vi "example.vi"() -> ()   [LabVIEW 2021]
uses:
  QR Code Reader.lvclass
  C:/Users/HEP/Documents/GitHub/Gantry/UCSB-Gantry-HEP-main/Classes/Controller/Camera/Camera.lvclass
  <vilib>/vision/Image Controls.llb/IMAQ Image.ctl
  <vilib>/vision/Instrument.llb/Data Matrix Report.ctl
  <vilib>/vision/Instrument.llb/ECC Type.ctl
  <vilib>/vision/Instrument.llb/Data Matrix Polarity.ctl
  <vilib>/vision/Instrument.llb/Cell Fill Percentage.ctl
  <vilib>/vision/Instrument.llb/Demodulation Mode.ctl
  <vilib>/vision/Instrument.llb/Cell Sample Size.ctl
  <vilib>/vision/Instrument.llb/Cell Filter Mode.ctl
  Camera.lvclass
panel:
  out "Data":string
  out "Barcode Report (2D Barcode Reader 1)":T1={"Found?"=FALSE, "Binary?"=FALSE, "Data"="", "Bounding Box"=[], "Errors Corrected"=0, "Erasures Corrected"=0, "Aspect Ratio"=0.0, "Rows"=0, "Columns"=0, "ECC"=-2, "Barcode Polarity"=-2, "Cell Fill Percentage"=-2, "Border Integrity"=0.0, "Mirrored?"=FALSE, "Minimum Edge Strength"=0, "Demodulation Mode"=-2, "Cell Sample Size"=-2, "Cell Filter Mode"=-2, "Iterations"=0} {"Barcode Polarity" items=["Auto-detect"=-2, "Black on White"=0, "White on Black"=1]; "Cell Fill Percentage" items=["Auto-detect"=-2, "< 30%"=0, ">= 30%"=1]; "Demodulation Mode" items=["Auto-detect"=-2, "Histogram"=0, "Local Contrast"=1, "Combination"=2, "All"=3]; "Cell Sample Size" items=["Auto-detect"=-2, "1x1"=1, "2x2"=2, "3x3"=3, "4x4"=4, "5x5"=5, "6x6"=6, "7x7"=7]; "Cell Filter Mode" items=["Auto-detect"=-2, "Average"=0, "Median"=1, "Central Avergae"=2, "High Average"=3, "Low Average"=4, "Very High Average"=5, "Very Low Average"=6, "All Filters"=8]; "ECC" items=["Auto-detect"=-2, "ECC 000"=0, "ECC 050"=50, "ECC 080"=80, "ECC 100"=100, "ECC 140"=140, "ECC 000-140"=190, "ECC 200"=200]; "Aspect Ratio" format="%.2f"; "Border Integrity" format="%_2f"; "Bounding Box"."y" format="%.2f"; "Bounding Box"."x" format="%.2f"}
  out "Image":T8(plugin-control)
  out "error out":errorcluster
  in  "error in (no error)":errorcluster
  out "Image Dst Out":T8
  out "QR Code Reader.lvclass":refnum<class "QR Code Reader.lvclass">
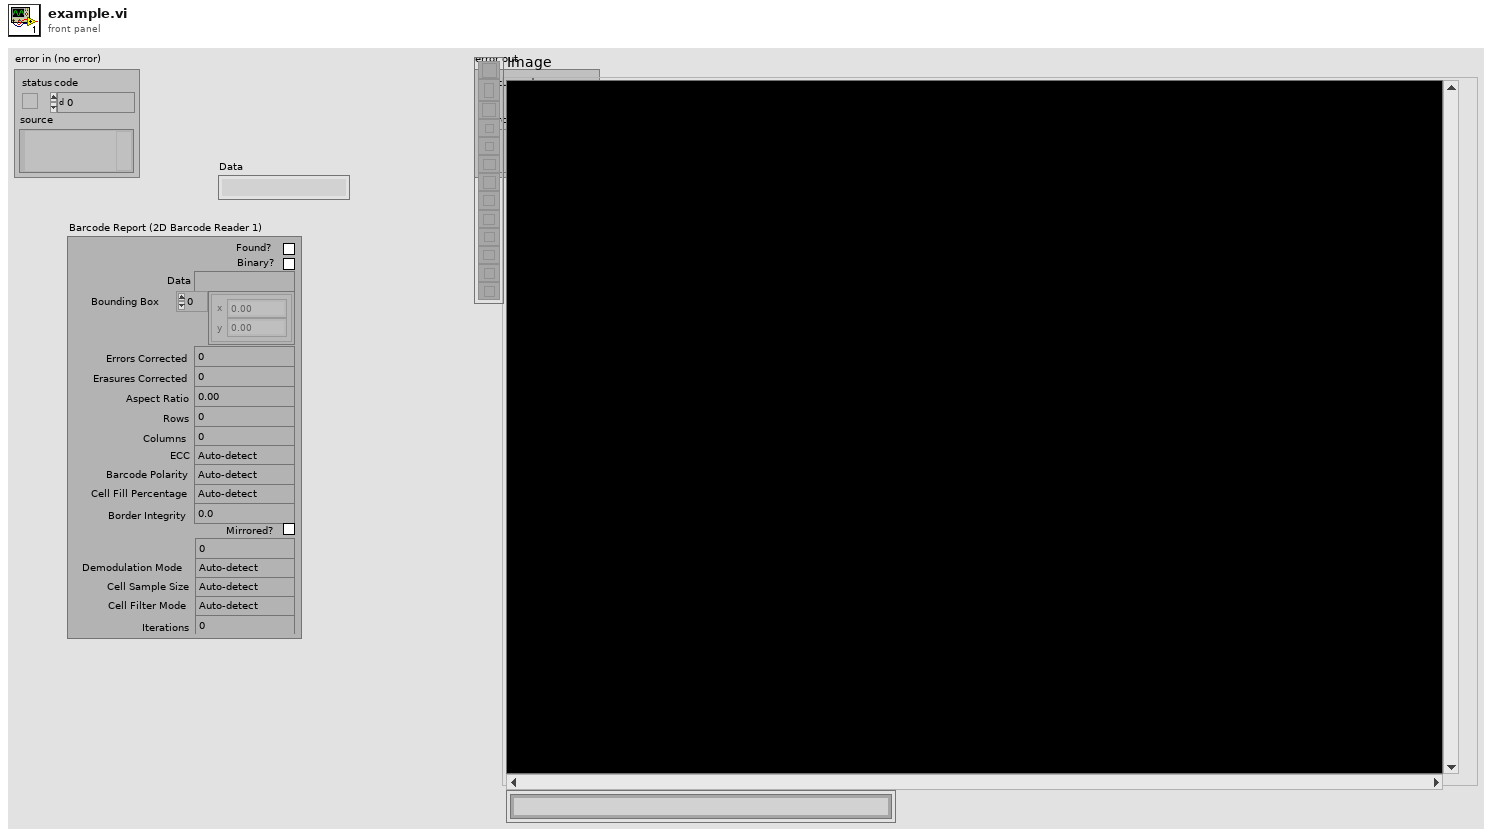
[diagram p1: front panel]
types:
  T1 = typedef "Data Matrix Report.ctl" = cluster{"Found?":bool, "Binary?":bool, "Data":string, "Bounding Box":cluster{"x":sgl, "y":sgl}[], "Errors Corrected":u32, "Erasures Corrected":u32, "Aspect Ratio":sgl, "Rows":u32, "Columns":u32, "ECC":T2, "Barcode Polarity":T3, "Cell Fill Percentage":T4, "Border Integrity":sgl, "Mirrored?":bool, "Minimum Edge Strength":u32, "Demodulation Mode":T5, "Cell Sample Size":T6, "Cell Filter Mode":T7, "Iterations":u32}
  T2 = typedef "ECC Type.ctl" = i32
  T3 = typedef "Data Matrix Polarity.ctl" = i32
  T4 = typedef "Cell Fill Percentage.ctl" = i32
  T5 = typedef "Demodulation Mode.ctl" = i32
  T6 = typedef "Cell Sample Size.ctl" = i32
  T7 = typedef "Cell Filter Mode.ctl" = i32
  T8 = typedef "IMAQ Image.ctl" = refnum<image>
  T9 = typedef "Image Type" = u32
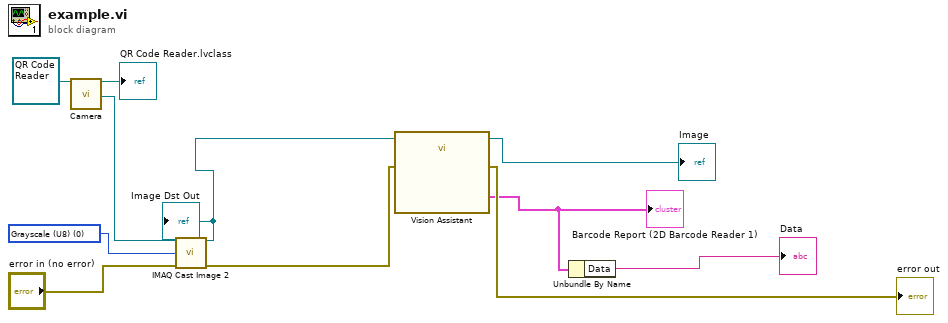
[diagram p0: block diagram]
diagram:
  w8 = T9 0 items=["Grayscale (U8)", "Grayscale (I16)", "Grayscale (SGL)", "Complex (CSG)", "RGB (U32)", "HSL (U32)", "RGB (U64)", "Grayscale (U16)"] ("Image Type")
  n1 = call "Camera.vi"("Camera in"=refnum<class "QR Code Reader.lvclass"> refnum ("QR Code Reader.lvclass")) -> ("Camera out"=→"QR Code Reader.lvclass":refnum<class "QR Code Reader.lvclass">, "Image"=w9:T8)  [unwired: 12 in, 5 out]
  n2 = call "IMAQ Cast Image 2"("Image Src"=w9, "Image Type"=w8, "error in (no error)"="error in (no error)") -> ("Image Dst Out"=w6:T8, "error out"=w4:errorcluster)  [unwired: 11 in]
  "Image Dst Out" <- w6
  n3 = call "Vision Assistant"("Image In"=w6, "error in"=w4) -> ("Image Out"=→"Image":T8, "Barcode Report (2D Barcode Reader 1)"=w2:T1, "error out"=→"error out":errorcluster)  [unwired: 23 in]
  "Barcode Report (2D Barcode Reader 1)" <- w2
  n4 = Unbundle By Name(w2) -> ("Data"=→"Data":string)
